vi "色阶计算.vi"(0 "多个颜色盒":u32[](array[colorbox]), 3 "阶数":i32=500) -> (14 "色阶":u32[](array[colorbox]))   [LabVIEW 2016]
uses:
  <vilib>/Analysis/1siggen.llb/Ramp Pattern by Samples.vi
  <vilib>/Analysis/NI_AALBase.lvlib
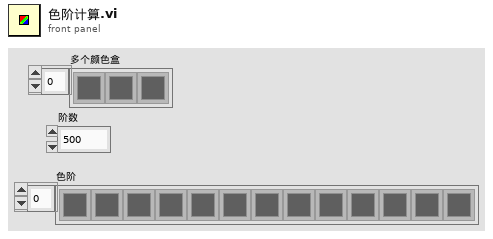
[diagram p1: front panel]
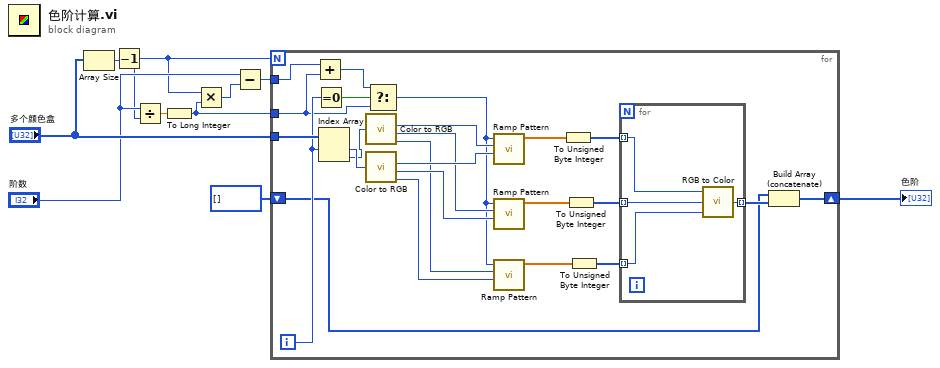
[diagram p0: block diagram]
diagram:
  n1 = Array Size(array="多个颜色盒") -> (size(s)=w1:i32)
  n2 = Decrement(x=w1) -> (x-1=w2:i32)
  n3 = Divide(x="阶数", y=w2) -> (x/y=w3:dbl)
  n4 = To Long Integer(number=w3) -> (32bit integer=w6:i32)
  n5 = Multiply(x=w2, y=w6) -> (x*y=w4:i32)
  n6 = Subtract(x="阶数", y=w4) -> (x-y=w7:i32)
  n7 = for {
    N: w2 -> [_]
    tunnel: "多个颜色盒" -> [w34]
    tunnel: w6 -> [w18]
    tunnel: w7 -> [w17]
    shift-right: [w14] -> w10
    shift-left: u32[] [] -> [w13]
    i -> [w20]
    n8 = Add(x=w17, y=w18) -> (x+y=w16:i32)
    n9 = Equal To 0?(x=w20) -> (x = 0?=w19:bool)
    n10 = Index Array(array=w34, index #1=w20) -> (element #1=w12:u32, element #2=w11:u32)  [unwired: 1 in]
    n11 = call <vilib>:"Color to RGB.vi"("Color"=w11) -> ("R"=w33:u8, "G"=w31:u8, "B"=w29:u8)  [unwired: 1 out]
    n12 = call <vilib>:"Color to RGB.vi"("Color"=w12) -> ("R"=w32:u8, "G"=w30:u8, "B"=w28:u8)  [unwired: 1 out]
    n13 = Select(t=w16, s=w19, f=w18) -> (s? t:f=w15:i32)
    n14 = call-poly <vilib>:"Ramp Pattern.vi"("start"=w32, "end"=w33, "samples"=w15) -> ("Ramp Pattern"=w27:dbl[])  [unwired: 7 in, 1 out]
    n15 = call-poly <vilib>:"Ramp Pattern.vi"("start"=w30, "end"=w31, "samples"=w15) -> ("Ramp Pattern"=w26:dbl[])  [unwired: 7 in, 1 out]
    n16 = call-poly <vilib>:"Ramp Pattern.vi"("start"=w28, "end"=w29, "samples"=w15) -> ("Ramp Pattern"=w25:dbl[])  [unwired: 7 in, 1 out]
    n17 = To Unsigned Byte Integer(number=w27) -> (unsigned 8bit integer=w24:u8[])
    n18 = To Unsigned Byte Integer(number=w26) -> (unsigned 8bit integer=w23:u8[])
    n19 = To Unsigned Byte Integer(number=w25) -> (unsigned 8bit integer=w22:u8[])
    n20 = for {
      tunnel: w24 -> [w38] mode=indexing
      tunnel: w23 -> [w37] mode=indexing
      tunnel: w22 -> [w36] mode=indexing
      tunnel: [w35] -> w21 mode=indexing
      n21 = call <vilib>:"RGB to Color.vi"("B"=w36, "G"=w37, "R"=w38) -> ("Color"=w35:u32)
    }
    n22 = Build Array (concatenate)(w13, w21) -> (w14:u32[])
  }
  "色阶" <- w10
